vi "WLAN_RSMA_FrameBuild.vi"(7 "Alpha":dbl min=0.0 max=1.0 step=0.05 format="%#_13g", 8 "error in (no error)":errorcluster, 9 "data in 2":i8[](array[numeric]) caption="input bit stream", 10 "Modulation parameter":T1, 11 "data in":i8[](array[numeric]) caption="input bit stream") -> (0 "error out":errorcluster, 3 "output array":cdb[](array[numeric]))   [LabVIEW 2022 SP3]
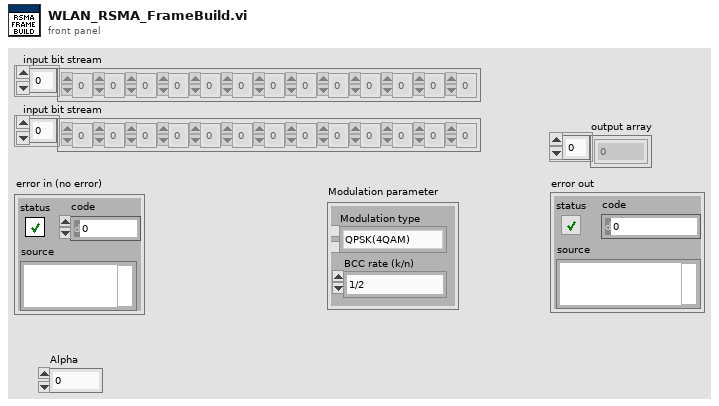
[diagram p1: front panel]
types:
  T1 = cluster{"Modulation type":enum16{"QPSK(4QAM)", "64QAM", "16QAM", "BPSK"}, "BCC rate (k/n)":enum16{"1/2", "2/3", "3/4"}}
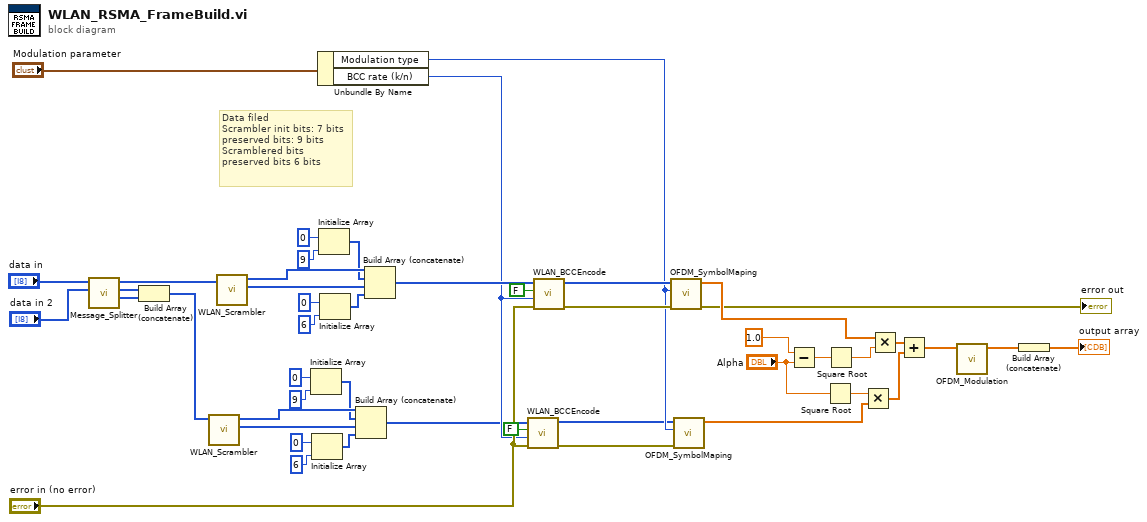
[diagram p0: block diagram]
diagram:
  # "Data filed\nScrambler init bits: 7 bits\npreserved bits: 9 bits\nScramblered bits\npreserved bits 6 bits"
  n1 = call "Message_Splitter.vi"("W2"="data in 2", "W1"="data in") -> ("Wp2"=w3:u8[], "Wp1"=w4:u8[], "Wc"=w2:u8[])  [unwired: 7 in]
  n2 = Build Array (concatenate)(w4, w3) -> (w1:u8[])
  n3 = call "WLAN_Scrambler.vi"("input bit stream"=w1) -> ("scrambled bits"=w22:i8[], "scrambler initial bit"=w26:i8[])  [unwired: 9 in]
  n4 = call "WLAN_Scrambler.vi"("input bit stream"=w2) -> ("scrambled bits"=w18:i8[], "scrambler initial bit"=w33:i8[])  [unwired: 9 in]
  n5 = Initialize Array(i8 0 ("element"), 9 ("dimension size")) -> (w25:i8[])
  n6 = Initialize Array(i8 0 ("element"), 6 ("dimension size")) -> (w19:i8[])
  n7 = Unbundle By Name("Modulation parameter") -> ("Modulation type"=w42:enum16{"QPSK(4QAM)", "64QAM", "16QAM", "BPSK"}, "BCC rate (k/n)"=w41:enum16{"1/2", "2/3", "3/4"})
  n8 = Initialize Array(i8 0 ("element"), 9 ("dimension size")) -> (w32:i8[])
  n9 = Initialize Array(i8 0 ("element"), 6 ("dimension size")) -> (w27:i8[])
  n10 = Build Array (concatenate)(w26, w25, w22, w19) -> (w38:i8[])
  n11 = Build Array (concatenate)(w33, w32, w18, w27) -> (w47:i8[])
  n12 = call "WLAN_BCCEncode.vi"("error in (no error)"="error in (no error)", "BCC rate (k/n)"=w41, "need add zeros?"=FALSE, "input bit stream"=w38) -> ("error out"=w36:errorcluster, "output bit stream 3"=w37:i8[])  [unwired: 6 in]
  n13 = call "WLAN_BCCEncode.vi"("error in (no error)"="error in (no error)", "BCC rate (k/n)"=w41, "need add zeros?"=FALSE, "input bit stream"=w47) -> ("error out"=w45:errorcluster, "output bit stream 3"=w44:i8[])  [unwired: 6 in]
  n14 = call "OFDM_SymbolMaping.vi"("error in (no error)"=w45, "Modulation type"=w42, "input bit stream"=w44) -> ("error out"=→"error out":errorcluster, "symbols"=w40:cdb[])  [unwired: 7 in]
  n15 = call "OFDM_SymbolMaping.vi"("error in (no error)"=w36, "Modulation type"=w42, "input bit stream"=w37) -> ("symbols"=w35:cdb[])  [unwired: 7 in, 1 out]
  n16 = Subtract(x=1.0, y="Alpha") -> (x-y=w10:dbl)
  n17 = Square Root(x="Alpha") -> (sqrt(x)=w14:dbl)
  n18 = Square Root(x=w10) -> (sqrt(x)=w12:dbl)
  n19 = Multiply(x=w14, y=w35) -> (x*y=w15:cdb[])
  n20 = Multiply(x=w40, y=w12) -> (x*y=w13:cdb[])
  n21 = Add(x=w13, y=w15) -> (x+y=w8:cdb[])
  n22 = call "OFDM_Modulation.vi"("Input sequence"=w8) -> ("Output sequence"=w7:cdb[])  [unwired: 10 in]
  n23 = Build Array (concatenate)(w7) -> (→"output array":cdb[])
